vi "StateMachineLocalDataAndErrorHandling.vi"() -> ()   [LabVIEW 2020]
uses:
  States.ctl
  <vilib>/ErrorRing/Error Ring.xnode
panel:
  out "Count":u32
  in  "Increment Counter":bool
  in  "stop":bool
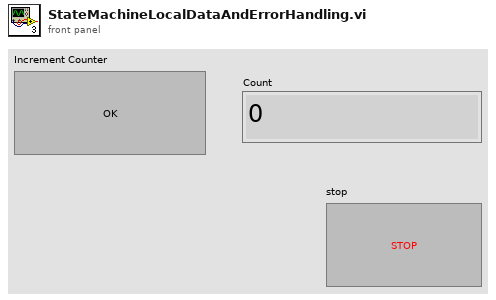
[diagram p1: front panel]
types:
  T1 = typedef "States.ctl" = enum16{"Idle", "Initialize", "IncrementNumber", "UpdateUI", "Process2", "Exit"}
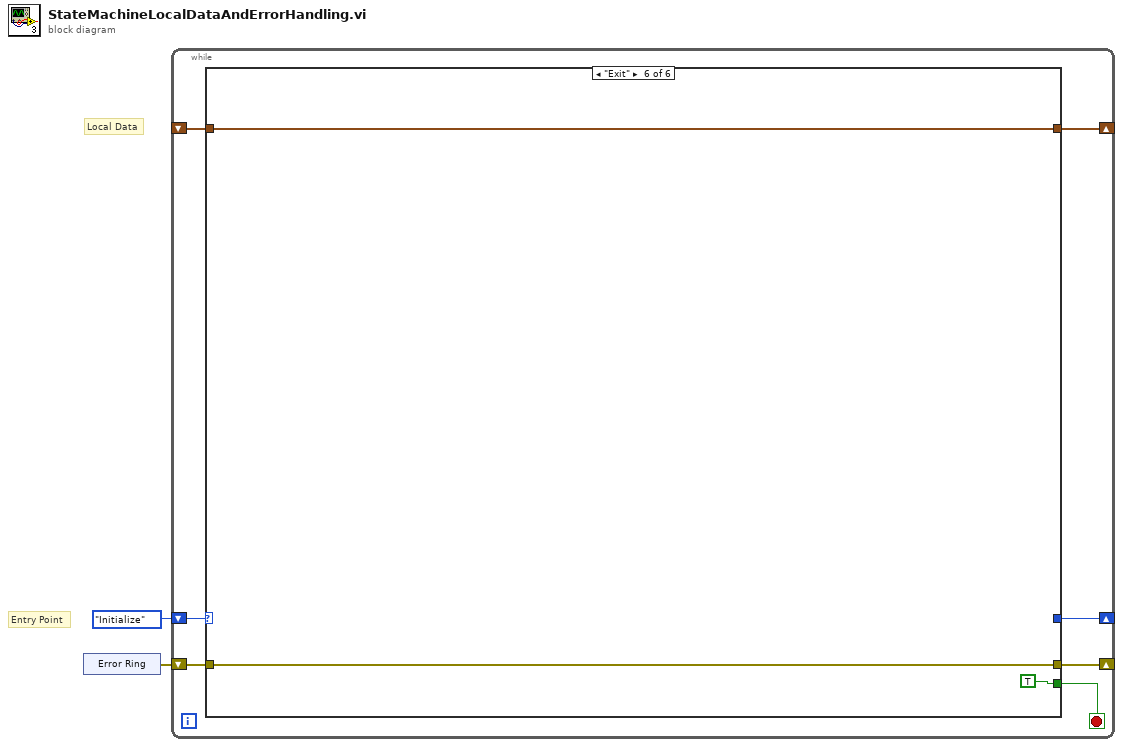
[diagram p0: block diagram]
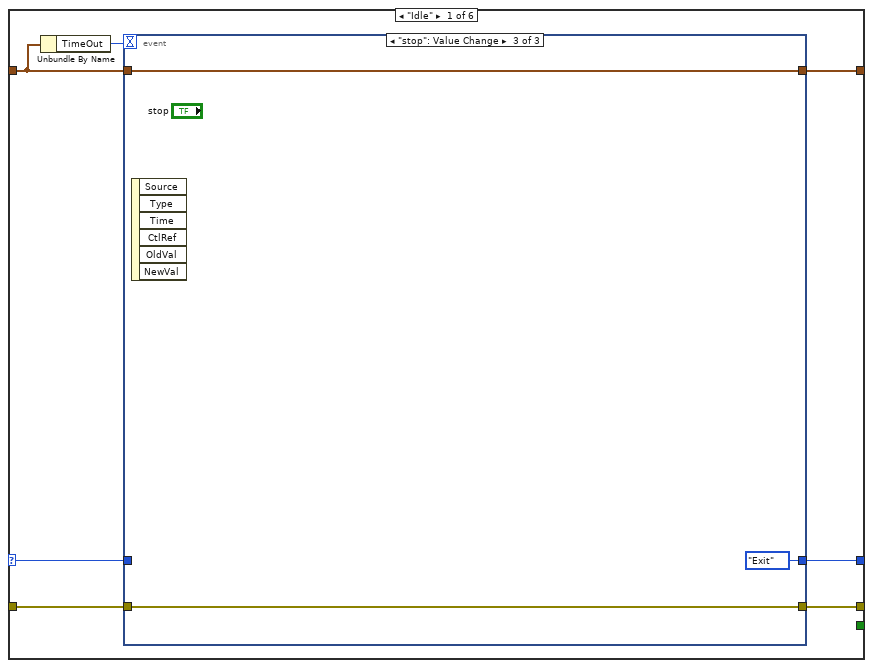
[diagram p2: hidden frame]
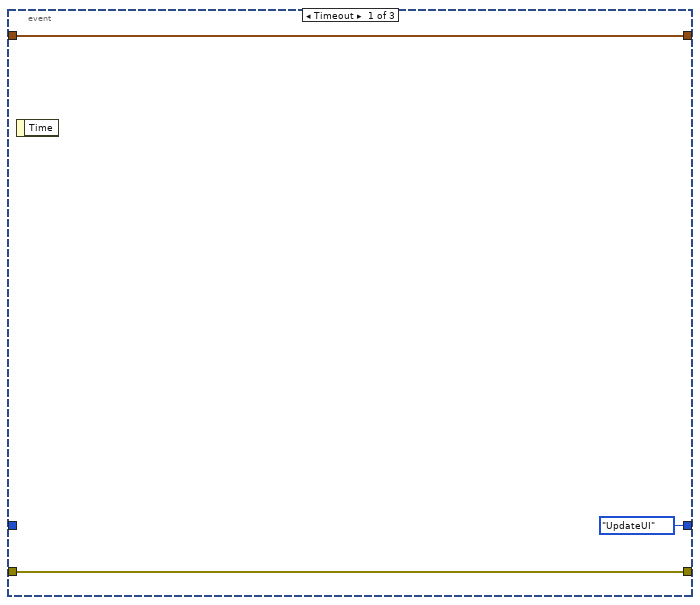
[diagram p3: hidden frame]
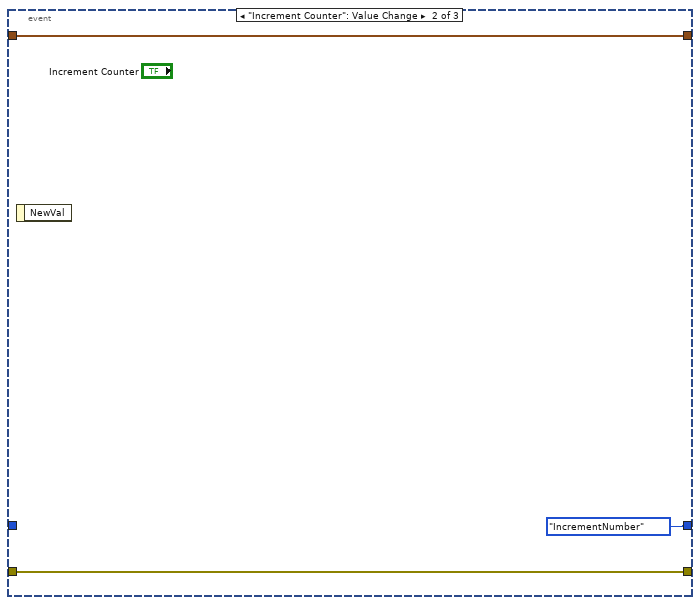
[diagram p4: hidden frame]
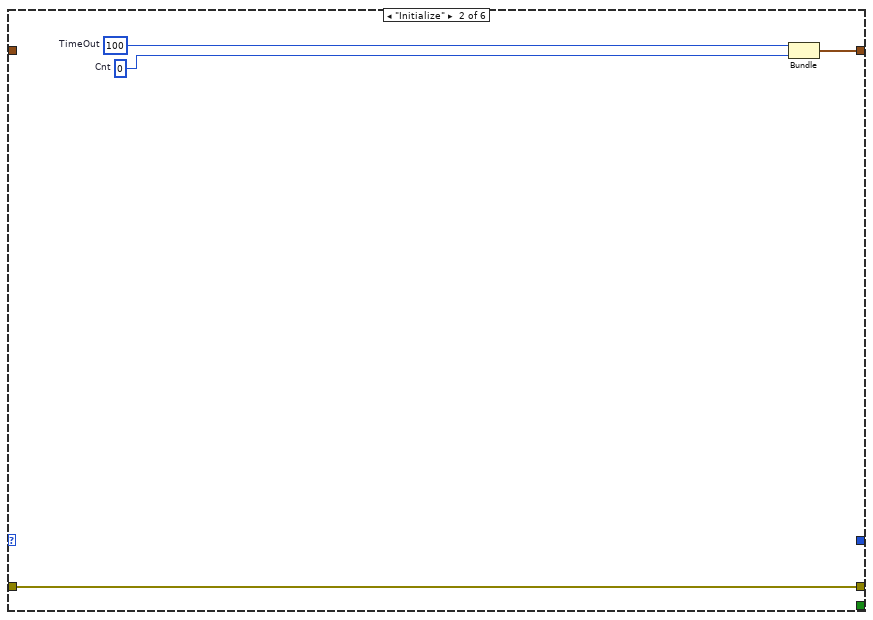
[diagram p5: hidden frame]
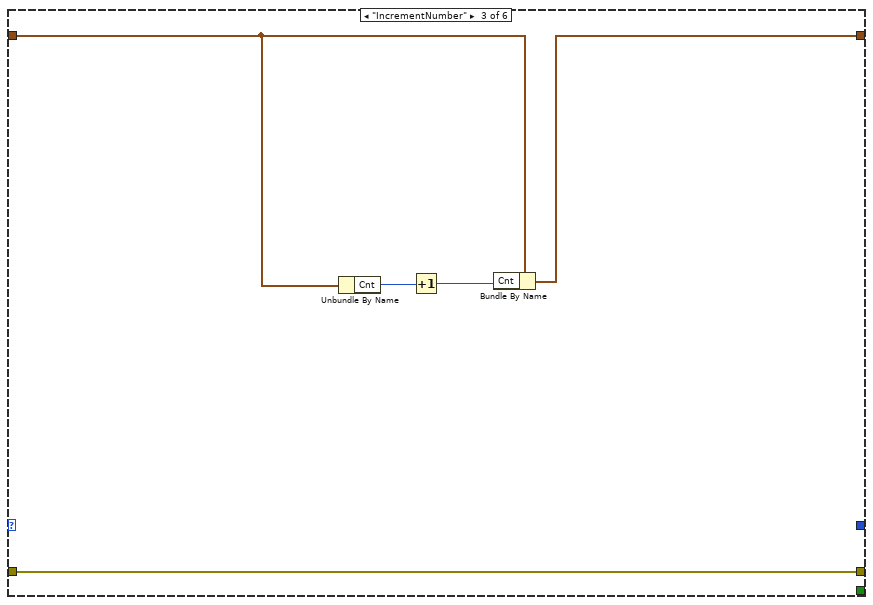
[diagram p6: hidden frame]
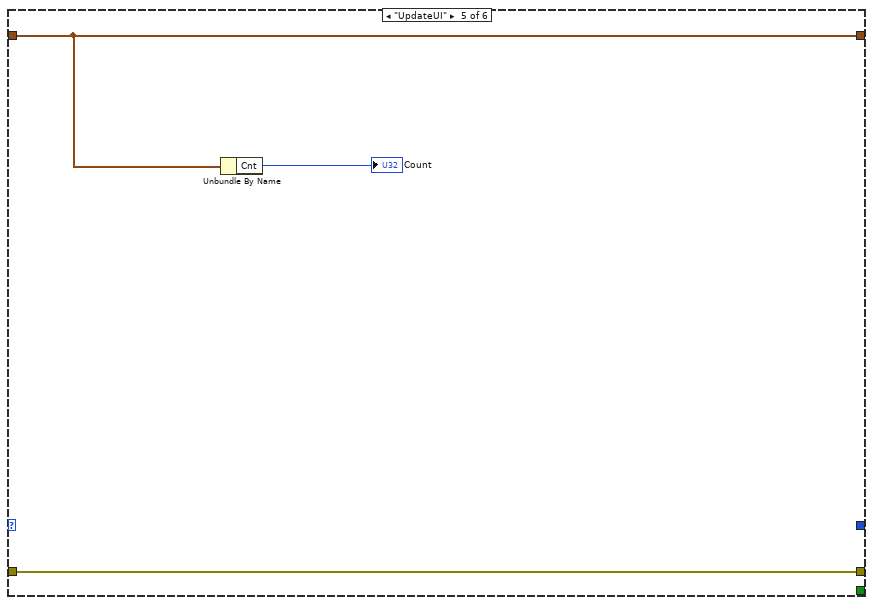
[diagram p8: hidden frame]
diagram:
  # "Local Data"
  # "Entry Point"
  n1 = xnode "Error Ring"() -> ("error out"=w1:errorcluster)
  n2 = while {
    shift-right: [w8] -> _
    shift-left: States."Initialize" -> [w9]
    shift-right: [w6] -> _
    shift-left: _ -> [w5]
    shift-right: [w3] -> _
    shift-left: w1 -> [w4]
    stop <- w7 stop-if-true
    n3 = case shown="\"Exit\"" w9 {
      selector: w9 -> [w16 _ _ _ _ _]
      tunnel: [w15 _ _ _ _ _] -> w8
      tunnel: [_ _ _ _ _ TRUE] -> w7
      tunnel: [w14 w29 w31 w36 w38 w41] -> w6
      tunnel: w5 -> [w11 _ w30 w36 w38 w41]
      tunnel: w4 -> [w13 w26 w34 w35 w39 w40]
      tunnel: [w12 w26 w34 w35 w39 w40] -> w3
      frame "Idle" {
        n4 = Unbundle By Name(w11) -> ("TimeOut"=w10:i32)
        n5 = event shown="[2] \"stop\": Value Change" {
          selector: _ -> [_ _ _]
          dyn-events: _ -> [_ _ _]
          timeout: w10 -> [_ _ _]
          tunnel: w16 -> [_ _ _]
          tunnel: [States."UpdateUI" States."IncrementNumber" States."Exit"] -> w15
          tunnel: w11 -> [w19 w22 w24]
          tunnel: [w19 w22 w24] -> w14
          tunnel: w13 -> [w18 w21 w23]
          tunnel: [w18 w21 w23] -> w12
          event Timeout {
            n6 = event-data() -> ()  [unwired: 1 in, 1 out]
          }
          event "Increment Counter": Value Change {
            n7 = event-data() -> ()  [unwired: 1 in, 1 out]
          }
          event "stop": Value Change {
            n8 = event-data() -> ()  [unwired: 1 in, 6 out]
          }
        }
      }
      frame "Initialize" {
        w27 = u32 0  # Cnt
        w28 = 100  # TimeOut
        n9 = Bundle("TimeOut"=w28, "Cnt"=w27) -> (w29:cluster{"TimeOut":i32, "Cnt":u32})  [unwired: 1 in]
      }
      frame "IncrementNumber" {
        n10 = Unbundle By Name(w30) -> ("Cnt"=w33:u32)
        n11 = Increment(x=w33) -> (x+1=w32:u32)
        n12 = Bundle By Name(cluster=w30, "Cnt"=w32) -> (w31:cluster{"TimeOut":i32, "Cnt":u32})
      }
      frame "Process2" {
      }
      frame "UpdateUI" {
        n13 = Unbundle By Name(w38) -> ("Cnt"=→"Count":u32)
      }
      frame "Exit" {
      }
    }
  }
